vi "finite_state_machine_1.vi"() -> ()   [LabVIEW 2023]
panel:
  out "State2":dbl(slide) scale=0.0..10.0
  out "State1":dbl(slide) scale=0.0..10.0
  in  "Exit":bool
  in  "State2":bool
  in  "State1":bool
  out "States":T1(ring)
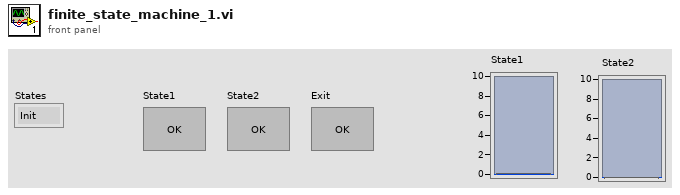
[diagram p1: front panel]
types:
  T1 = enum16{"Init", "Wait", "State1", "State2", "Exit"}
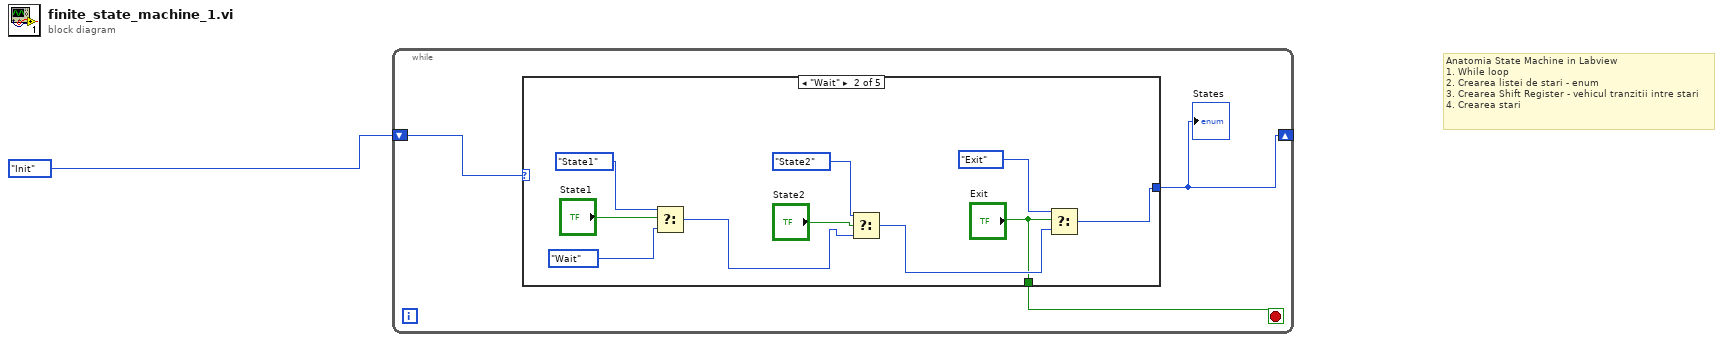
[diagram p0: block diagram]
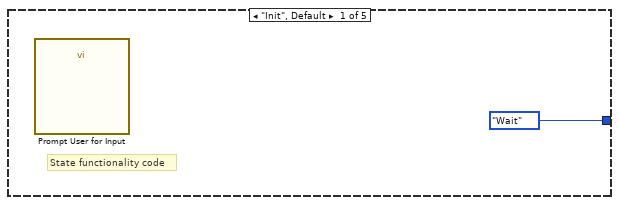
[diagram p2: hidden frame]
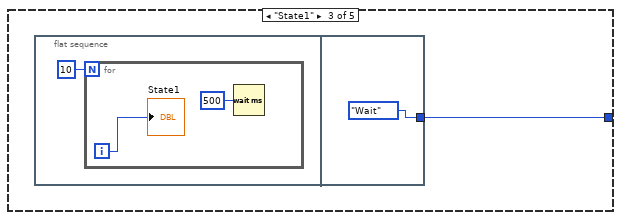
[diagram p3: hidden frame]
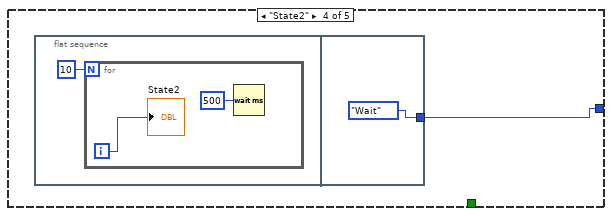
[diagram p4: hidden frame]
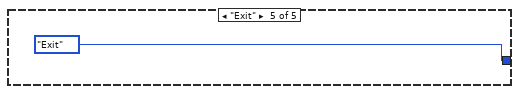
[diagram p5: hidden frame]
diagram:
  # "Anatomia State Machine in Labview\n1. While loop\n2. Crearea listei de stari - enum\n3. Crearea Shift Register - vehicul tranzitii intre stari\n4. Crearea stari"
  n1 = while {
    shift-right: [w2] -> _
    shift-left: T1."Init" ("States") -> [w4]
    stop <- w3 stop-if-true
    n2 = case shown="\"Wait\"" w4 {
      tunnel: [T1."Wait" ("States") w7 w16 w21 T1."Exit" ("States")] -> w2
      tunnel: [_ "Exit" _ _ _] -> w3
      frame "Init", Default {
        # "State functionality code"
        n3 = call "Prompt User for Input"() -> ()  [unwired: 18 in, 2 out]
      }
      frame "Wait" {
        n4 = Select(t=T1."State1" ("States"), s="State1", f=T1."Wait" ("States")) -> (s? t:f=w10:T1)
        n5 = Select(t=T1."State2" ("States"), s="State2", f=w10) -> (s? t:f=w8:T1)
        n6 = Select(t=T1."Exit" ("States"), s="Exit", f=w8) -> (s? t:f=w7:T1)
      }
      frame "State1" {
        n7 = flat-sequence {
          tunnel: [T1."Wait" ("States")] -> w16
          frame #0 {
            n8 = for {
              N: 10 -> [_]
              i -> [w19]
              n9 = Wait (ms)(milliseconds to wait=u32 500) -> ()  [unwired: 1 out]
              "State1" <- w19
            }
          }
          frame #1 {
          }
        }
      }
      frame "State2" {
        n10 = flat-sequence {
          tunnel: [T1."Wait" ("States")] -> w21
          frame #0 {
            n11 = for {
              N: 10 -> [_]
              i -> [w24]
              n12 = Wait (ms)(milliseconds to wait=u32 500) -> ()  [unwired: 1 out]
              "State2" <- w24
            }
          }
          frame #1 {
          }
        }
      }
      frame "Exit" {
      }
    }
    "States" <- w2
  }
